vi "nanostage-health.vi"(2 "error in":errorcluster, 3 "All conn. axes":string[](array[string])) -> (0 "error":bool, 1 "error message":string)   [LabVIEW 2015]
panel:
  out "z-axis":bool
  out "x-axis":bool
  out "y-axis":bool
  # "3D piezo nano stage"
  # "closed loop active?"
  # "status x-axis"
  # "status y-axis"
  # "status z-axis"
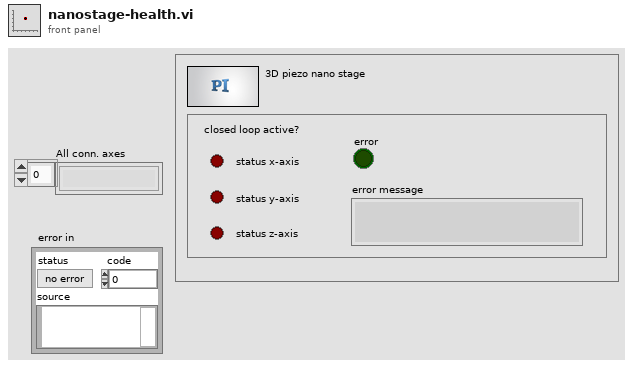
[diagram p1: front panel]
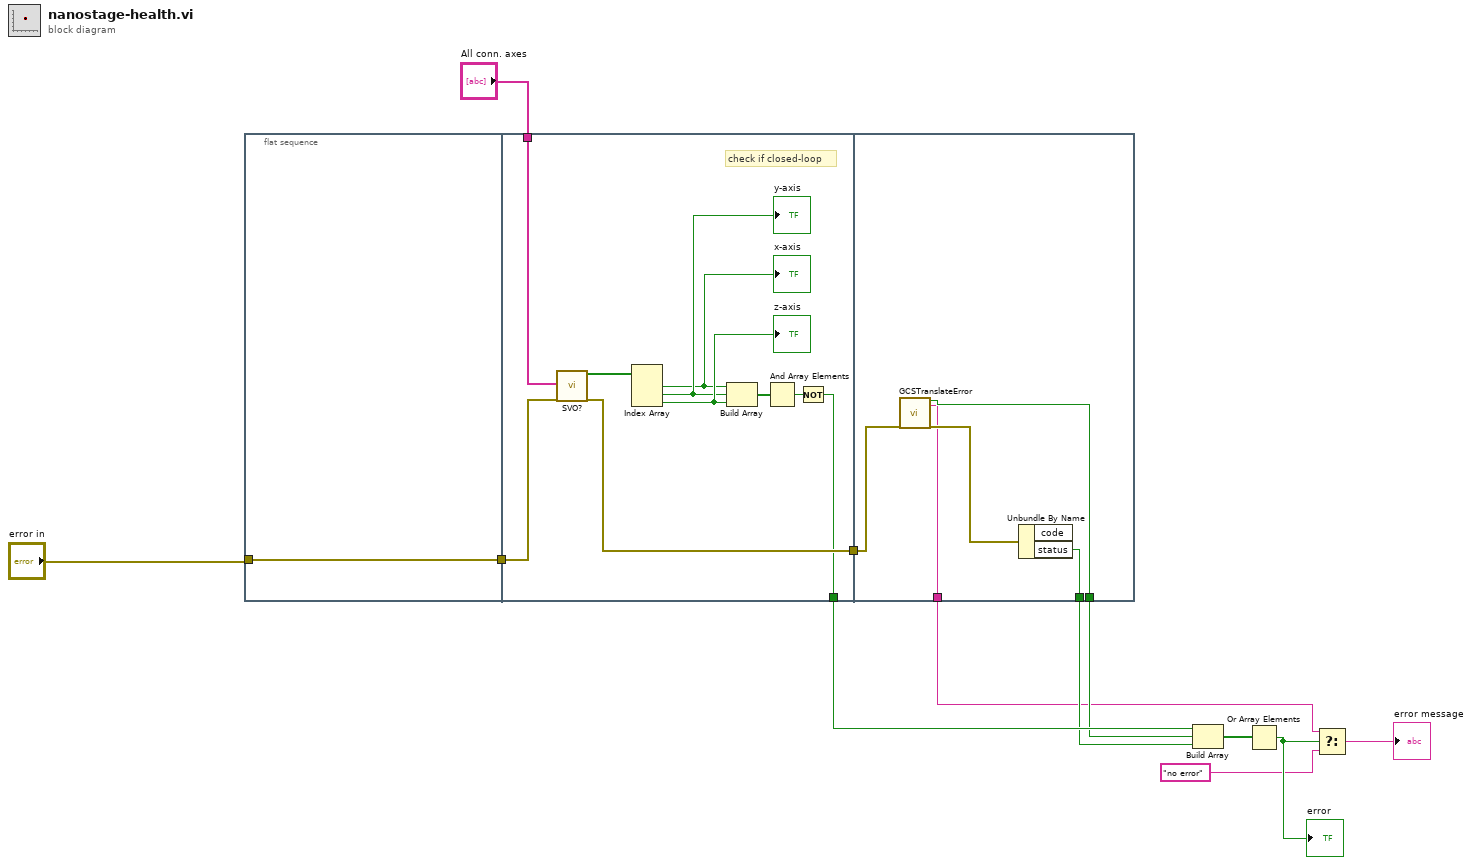
[diagram p0: block diagram]
diagram:
  n1 = flat-sequence {
    tunnel: "error in" -> [w13]
    tunnel: [w13] -> w11
    tunnel: w11 -> [w21]
    tunnel: "All conn. axes" -> [w20]
    tunnel: [w19] -> w9
    tunnel: [w14] -> w8
    tunnel: w9 -> [w27]
    tunnel: [w26] -> w4
    tunnel: [w25] -> w3
    tunnel: [w24] -> w2
    frame #0 {
    }
    frame #1 {
      # "check if closed-loop"
      n2 = call "SVO?.vi"("Axes to query"=w20, "error in"=w21) -> ("Servo status?"=w23:bool[], "error out"=w19:errorcluster)  [unwired: 16 in]
      n3 = Index Array(array=w23) -> (element #1=w16:bool, element #2=w17:bool, element #3=w22:bool)  [unwired: 3 in]
      "y-axis" <- w17
      "x-axis" <- w16
      "z-axis" <- w22
      n4 = Build Array(w16, w17, w22) -> (w18:bool[])
      n5 = And Array Elements(Boolean array=w18) -> (logical AND=w15:bool)
      n6 = Not(x=w15) -> (.not. x?=w14:bool)
    }
    frame #2 {
      n7 = call "GCSTranslateError.vi"("error in"=w27) -> ("GCS Error?"=w25:bool, "Error Description"=w24:string, "error out"=w28:errorcluster)  [unwired: 16 in]
      n8 = Unbundle By Name(w28) -> ("status"=w26:bool)  [unwired: 1 out]
    }
  }
  n9 = Build Array(w8, w3, w4) -> (w7:bool[])
  n10 = Or Array Elements(Boolean array=w7) -> (logical OR=w6:bool)
  "error" <- w6
  n11 = Select(t=w2, s=w6, f="no error" ("t")) -> (s? t:f=→"error message":string)
